vi "Fpga_v7.vi"() -> ()   [LabVIEW 2015]
uses:
  <vilib>/Platform/TimedLoop/XDataNode/timing_clust.ctl
  <vilib>/Platform/TimedLoop/XDataNode/nitl_modes.ctl
  <vilib>/Platform/TimedLoop/XDataNode/wakeup.ctl
  <vilib>/rvi/Emulation/niFpgaGetClockAttributes.vi
  <vilib>/rvi/Emulation/niFpgaSctlEmulationGetInTimedLoop.vi
  <vilib>/rvi/Emulation/niFpgaEmulationReportErrorSimple.vi
  <vilib>/rvi/eio/common/nirviEmuTemplateMethod_errors.vi
  <vilib>/rvi/Emulation/niFpgaCriticalErrorInLSC.vi
  <vilib>/rvi/occurrence/nirviWaitOnOccurrenceBase.vi
  <vilib>/rvi/Emulation/niFpgaProcessEmulError.vi
  <vilib>/eio/EIONode/EIONode.xnode
  <vilib>/Platform/TimedLoop/XDataNode/XDataNode.xnode
  <vilib>/Platform/TimedLoop/XDataNode/XDNodeRunTimeDep.lvlib
panel:
  out "Gauge":i16(knob) scale=0.0..20000.0
  out "x-y":u32
  out "Encoder data in 8":bool
  out "Aquisition loop rate":u32
  out "Data aqusitioning 2":bool
  out "Encoder data in 7":bool
  out "Encoder data in 6":bool
  out "Encoder data in 5":bool
  out "Encoder data in 4":bool
  out "Encoder data in 3":bool
  out "Encoder data in 2":bool
  out "Internal FPGA wiring works":bool
  in  "Mod4/AO0 2":i16
  out "Mod3/AI0 2":fxp<+/-,16,5>
  out "DI0 oN":bool
  out "Encoder data in":bool
  in  "Data write ON/OFF 2":bool
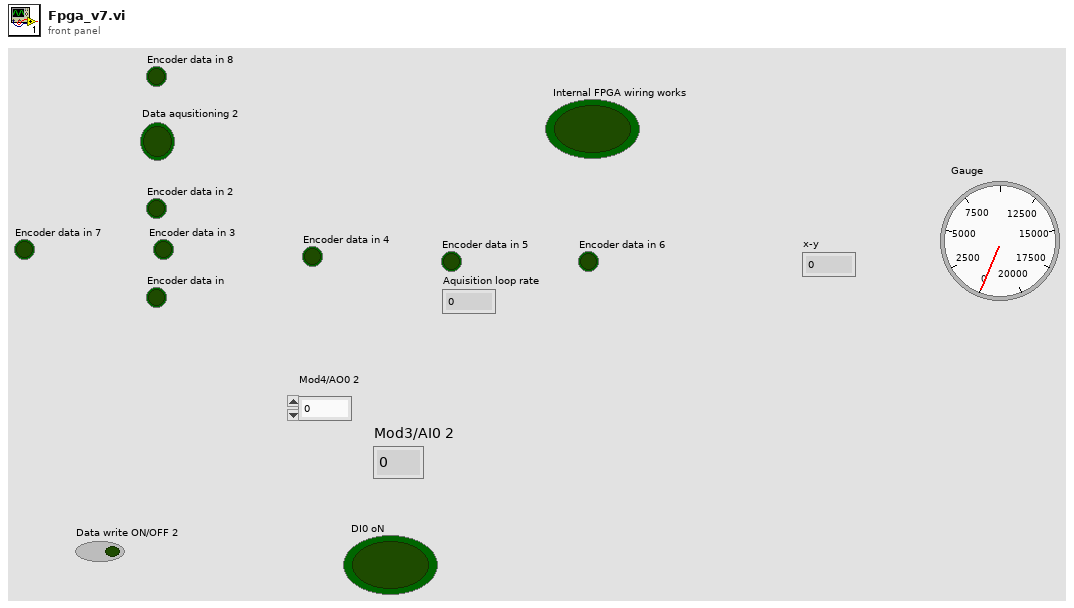
[diagram p1: front panel]
types:
  T1 = typedef "XDNodeRunTimeDep.lvlib/timing_clust.ctl" = cluster{"Expected End [f-1]":u64, "Actual End [f-1]":u64, "Finished Late? [f-1]":bool, "Expected End [i-1]":u64, "Actual End [i-1]":u64, "Finished Late? [i-1]":bool, "Expected Start [i]":u64, "Actual Start [i]":u64, "Expected Start [f]":u64, "Actual Start [f]":u64, "Source Name":string, "Structure Name":string, "Period":i64, "Deadline":i64, "Offset":i64, "Start":i64, "Priority":i32, "Timeout":i32, "Mode":T2, "Wakeup Reason":T3, "Error":errorcluster, "Source Type":string, "Secondary Source Type":string, "Global End Time":u64, "Global Start Time":u64, "Frame Duration":u64, "Iteration Duration":u64, "Assigned CPU":i32, "I/O Scan Engine Mode":u32}
  T2 = typedef "XDNodeRunTimeDep.lvlib/nitl_modes.ctl" = enum32{"No Change", "Process missed periods, maintain original phase", "Discard missed periods, maintain original phase", "Process missed periods, ignore original phase", "Discard missed periods, ignore original phase"}
  T3 = typedef "XDNodeRunTimeDep.lvlib/wakeup.ctl" = enum32{"Normal", "Aborted", "Asynchronous wakeup", "Timing source error", "Timed loop error", "Timeout"}
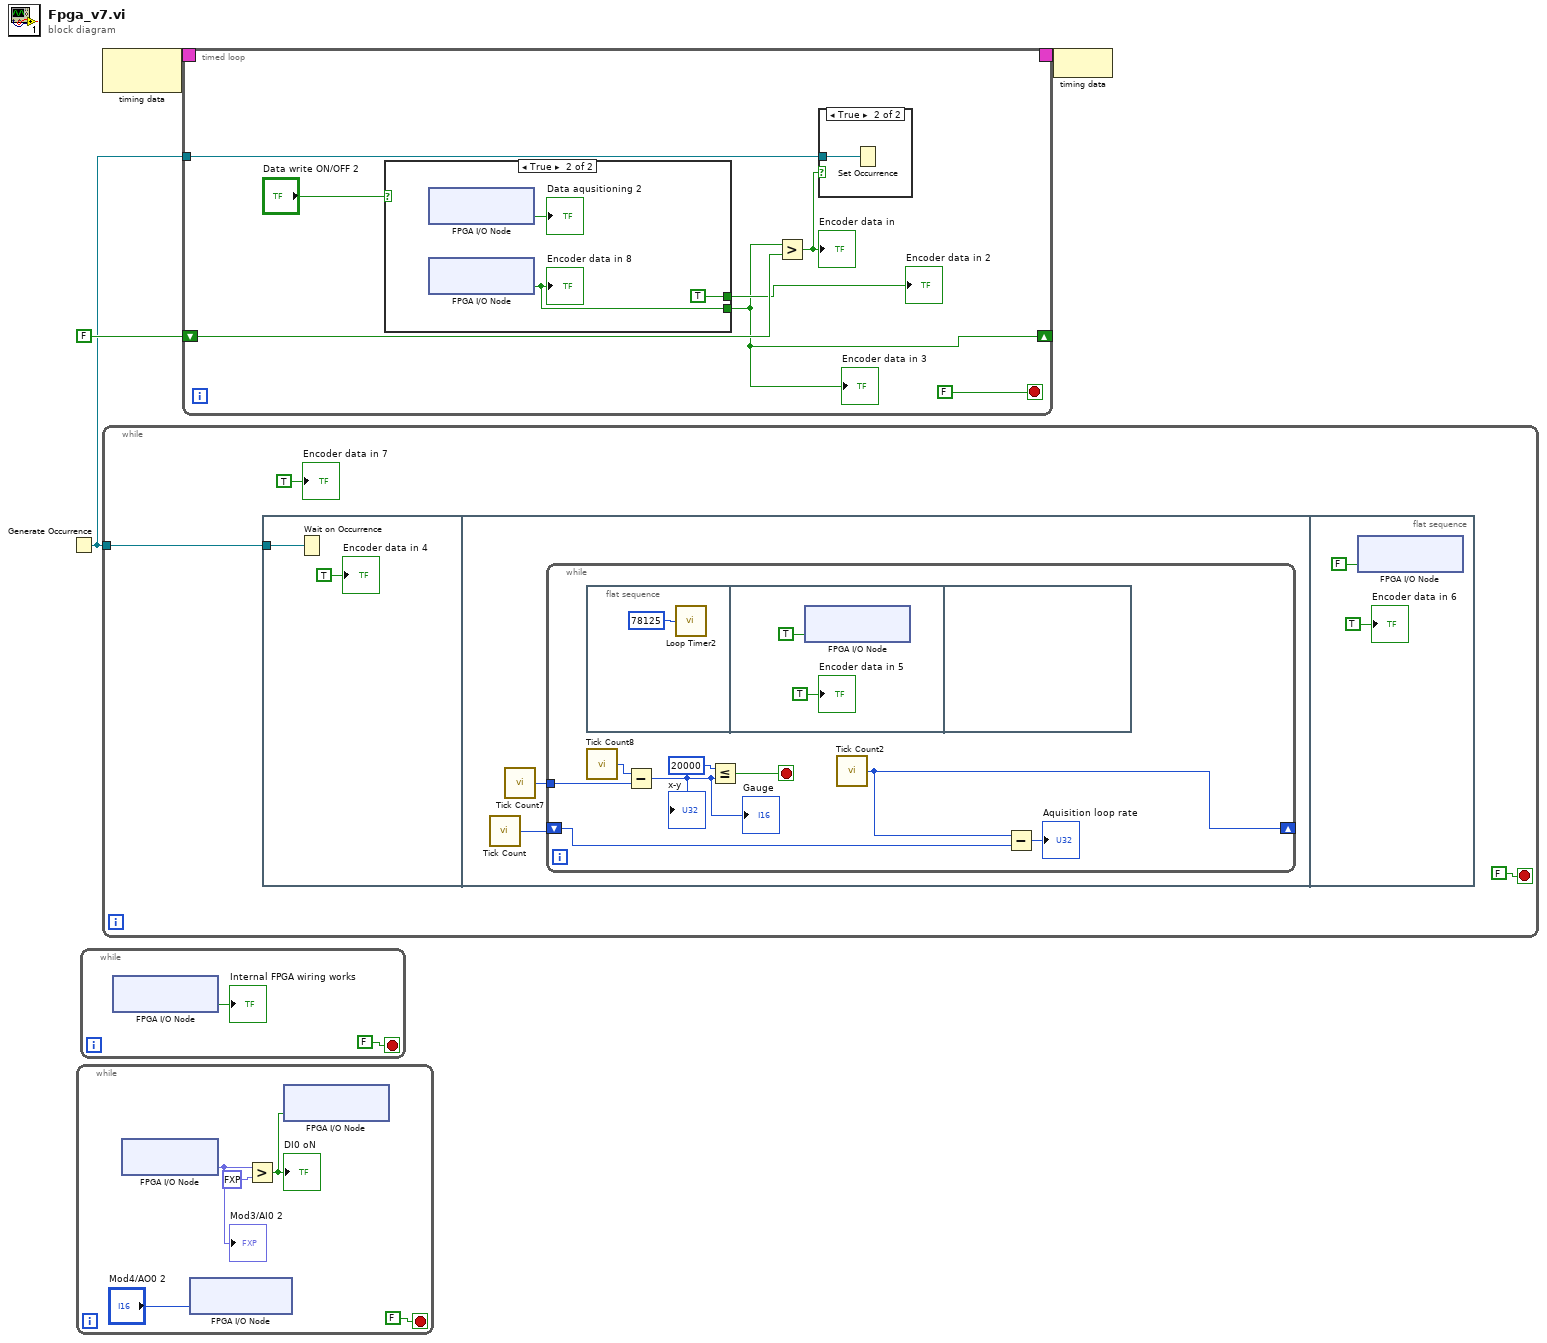
[diagram p0: block diagram]
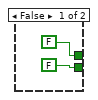
[diagram p3: hidden frame]
diagram:
  n1 = Generate Occurrence() -> (w1:refnum<k4>)
  n2 = while {
    stop <- FALSE stop-if-true
    n3 = xnode "FPGA I/O Node"() -> ("Mod3/AI0"=w6:fxp<+/-,16,5>)  [unwired: 1 in, 1 out]
    "Mod3/AI0 2" <- w6
    n4 = xnode "FPGA I/O Node"("Mod4/AO1"="Mod4/AO0 2") -> ()  [unwired: 1 in, 1 out]
    n5 = Greater?(x=w6, y=fxp<+/-,16,5> 2.0) -> (0:w5:bool)
    "DI0 oN" <- w5
    n6 = xnode "FPGA I/O Node"("Mod2/DIO0"=w5) -> ()  [unwired: 1 in, 1 out]
  }
  n7 = while {
    stop <- FALSE stop-if-true
    n8 = xnode "FPGA I/O Node"() -> ("Mod2/DIO0"=→"Internal FPGA wiring works":bool)  [unwired: 1 in, 1 out]
  }
  n9 = node-c288() -> (w4:T1)  [unwired: 1 in]
  n10 = while {
    tunnel: w1 -> [w13]
    stop <- FALSE stop-if-true
    n11 = flat-sequence {
      tunnel: w13 -> [w16]
      frame #0 {
        n12 = Wait on Occurrence(2:w16) -> ()  [unwired: 2 in, 1 out]
        "Encoder data in 4" <- TRUE ("Encoder data in 4")
      }
      frame #1 {
        n13 = call "Tick Count"() -> ("Tick Count(mSec)"=w17:u32)
        n14 = call "Tick Count7"() -> ("Tick Count(mSec)"=w18:u32)
        n15 = while {
          tunnel: w18 -> [w25]
          shift-right: [w20] -> _
          shift-left: w17 -> [w21]
          stop <- w23 stop-if-true
          n16 = flat-sequence {
            frame #0 {
              n17 = call "Loop Timer2"("Count(Ticks)"=u32 78125 ("Count(mSec)")) -> ()  [unwired: 1 out]
            }
            frame #1 {
              n18 = xnode "FPGA I/O Node"("Mod2/DIO7"=TRUE ("Boolean")) -> ()  [unwired: 1 in, 1 out]
              "Encoder data in 5" <- TRUE ("Encoder data in 4")
            }
            frame #2 {
            }
          }
          n19 = call "Tick Count8"() -> ("Tick Count(mSec)"=w26:u32)
          n20 = Subtract(x=w26, y=w25) -> (x-y=w19:u32)
          "x-y" <- w19
          "Gauge" <- w19
          n21 = Less Or Equal?(x=u32 20000, y=w19) -> (x <= y?=w23:bool)
          n22 = call "Tick Count2"() -> ("Tick Count(Ticks)"=w20:u32)
          n23 = Subtract(x=w20, y=w21) -> (x-y=→"Aquisition loop rate":u32)
        }
      }
      frame #2 {
        n24 = xnode "FPGA I/O Node"("Mod2/DIO7"=FALSE ("Boolean")) -> ()  [unwired: 1 in, 1 out]
        "Encoder data in 6" <- TRUE ("Encoder data in 4")
      }
    }
    "Encoder data in 7" <- TRUE ("Encoder data in 4")
  }
  n25 = timed-loop {
    timing: w4 -> [_]
    timing-out: [_] -> w3
    shift-right: [w33] -> _
    shift-left: FALSE -> [w37]
    tunnel: w1 -> [w36]
    stop <- FALSE stop-if-true
    n26 = case shown="True" "Data write ON/OFF 2" {
      tunnel: [FALSE ("Mod2/DIO6") w42] -> w33
      tunnel: [FALSE ("Encoder data in 2") TRUE ("Encoder data in 2")] -> w34
      frame False {
      }
      frame True {
        n27 = xnode "FPGA I/O Node"() -> ("Mod2/DIO6"=→"Data aqusitioning 2":bool)  [unwired: 1 in, 1 out]
        n28 = xnode "FPGA I/O Node"() -> ("Mod2/DIO2"=w42:bool)  [unwired: 1 in, 1 out]
        "Encoder data in 8" <- w42
      }
    }
    "Encoder data in 2" <- w34
    "Encoder data in 3" <- w33
    n29 = Greater?(x=w33, y=w37) -> (0:w32:bool)
    "Encoder data in" <- w32
    n30 = case shown="True" w32 {
      tunnel: w36 -> [_ w39]
      frame False {
      }
      frame True {
        n31 = Set Occurrence(w39) -> ()
      }
    }
  }
  n32 = node-c288(w3) -> ()
